vi "top_loop.vi"(0 "Input parameters":T4={"Measurement type"=enum."Debug", "Sensor type"=enum."HPK_8in_256", "Identifier"="test.txt", "Open after execution?"=FALSE, "Plot after execution?"=FALSE, "Display channel"=0, "Voltage Delay (s)"=0.5, "Switch Delay (s)"=0.01, "VISA resource name source"="", "VISA resource name DMM"="", "VISA resource name LCR"="", "Compliance  Level (A)"=10.0, "Voltage Limit (V)"=1000.0, "Data storage location"="", "Scan voltages"="", "Use source as DMM?"=FALSE, "LCR signal frequenzy (Hz)"=10.0, "DMM device"=enum."Keithley2001", "Sampling number"=1, "Use env. sensors on"=enum."Sensirion sht1x/7x", "Switchboard Handle"=0, "Use Switchboard"=FALSE, "LCR signal voltage (V)"=10000.0, "Repeat"=1, "Scan voltages IV"="", "Scan voltages CV"="", "Hex pad numbers?"=FALSE, "Set measurement type"=enum."Debug", "Custom pad scan"="", "IV voltage Delay (s)"=0.5, "CV voltage Delay (s)"=0.5, "Needle measurement?"=FALSE, "Comments"="test.txt", "LCR signal frequenzy (kHz)"=10.0, "Compliance  Level (uA)"=10.0, "Open Correction Array"=array2304x3[6912 elements], "Current set voltage"=0.0, "Last set voltage"=0.0, "Current channel"=0, "Last OpenCorrection index"=-1, "Total curr/vltg every x steps"=10, "Current channel iteration"=0, "No CV corrections"=FALSE, "Mapfile"="", "Corrfile"="", "IV voltage file"=path "", "CV voltage file"=path "", "IV Switch Delay (s)"=0.01, "CV Switch Delay (s)"=0.01, "Invert polarity"=FALSE, "Set debug dirs"=FALSE, "Is n on p"=FALSE} {"CV Switch Delay (s)" format="%#_13g"; "IV Switch Delay (s)" format="%#_13g"; "Last set voltage" format="%#_13g"; "Current set voltage" format="%#_13g"; "CV voltage Delay (s)" format="%#_13g"; "IV voltage Delay (s)" format="%#_13g"; "Voltage Limit (V)" format="%#_13g"; "Voltage Delay (s)" format="%#_13g"; "Switch Delay (s)" format="%#_13g"}, 5 "Dynamic data":T3, 7 "Front_panel_refs":T1, 11 "error in (no error)":errorcluster, 12 "Environmental data":T2) -> (4 "Input parameters out":T4={"Measurement type"=enum."Debug", "Sensor type"=enum."HPK_8in_256", "Identifier"="test.txt", "Open after execution?"=FALSE, "Plot after execution?"=FALSE, "Display channel"=0, "Voltage Delay (s)"=0.5, "Switch Delay (s)"=0.01, "VISA resource name source"="", "VISA resource name DMM"="", "VISA resource name LCR"="", "Compliance  Level (A)"=10.0, "Voltage Limit (V)"=1000.0, "Data storage location"="", "Scan voltages"="", "Use source as DMM?"=FALSE, "LCR signal frequenzy (Hz)"=10.0, "DMM device"=enum."Keithley2001", "Sampling number"=1, "Use env. sensors on"=enum."Sensirion sht1x/7x", "Switchboard Handle"=0, "Use Switchboard"=FALSE, "LCR signal voltage (V)"=10000.0, "Repeat"=1, "Scan voltages IV"="", "Scan voltages CV"="", "Hex pad numbers?"=FALSE, "Set measurement type"=enum."Debug", "Custom pad scan"="", "IV voltage Delay (s)"=0.5, "CV voltage Delay (s)"=0.5, "Needle measurement?"=FALSE, "Comments"="test.txt", "LCR signal frequenzy (kHz)"=10.0, "Compliance  Level (uA)"=10.0, "Open Correction Array"=array2304x3[6912 elements], "Current set voltage"=0.0, "Last set voltage"=0.0, "Current channel"=0, "Last OpenCorrection index"=-1, "Total curr/vltg every x steps"=10, "Current channel iteration"=0, "No CV corrections"=FALSE, "Mapfile"="", "Corrfile"="", "IV voltage file"=path "", "CV voltage file"=path "", "IV Switch Delay (s)"=0.01, "CV Switch Delay (s)"=0.01, "Invert polarity"=FALSE, "Set debug dirs"=FALSE, "Is n on p"=FALSE} {"CV Switch Delay (s)" format="%#_13g"; "IV Switch Delay (s)" format="%#_13g"; "Last set voltage" format="%#_13g"; "Current set voltage" format="%#_13g"; "CV voltage Delay (s)" format="%#_13g"; "IV voltage Delay (s)" format="%#_13g"; "Voltage Limit (V)" format="%#_13g"; "Voltage Delay (s)" format="%#_13g"; "Switch Delay (s)" format="%#_13g"}, 6 "Dynamic data out":T3, 8 "Front_panel_refs out":T1, 15 "error out":errorcluster)   [LabVIEW 2016]
doc: "The main loop function of the HexDAQ."
uses:
  <extravilib>/ChannelInstances/Tag-t'Env_data.ctl'.lvlib
  data_live.ctl
  input_params.ctl
  data_dynamic.ctl
  data_env.ctl
  <extravilib>/ChannelInstances/Tag-t'Env_data.ctl'/))Channel.ctl
  refs_front_panel.ctl
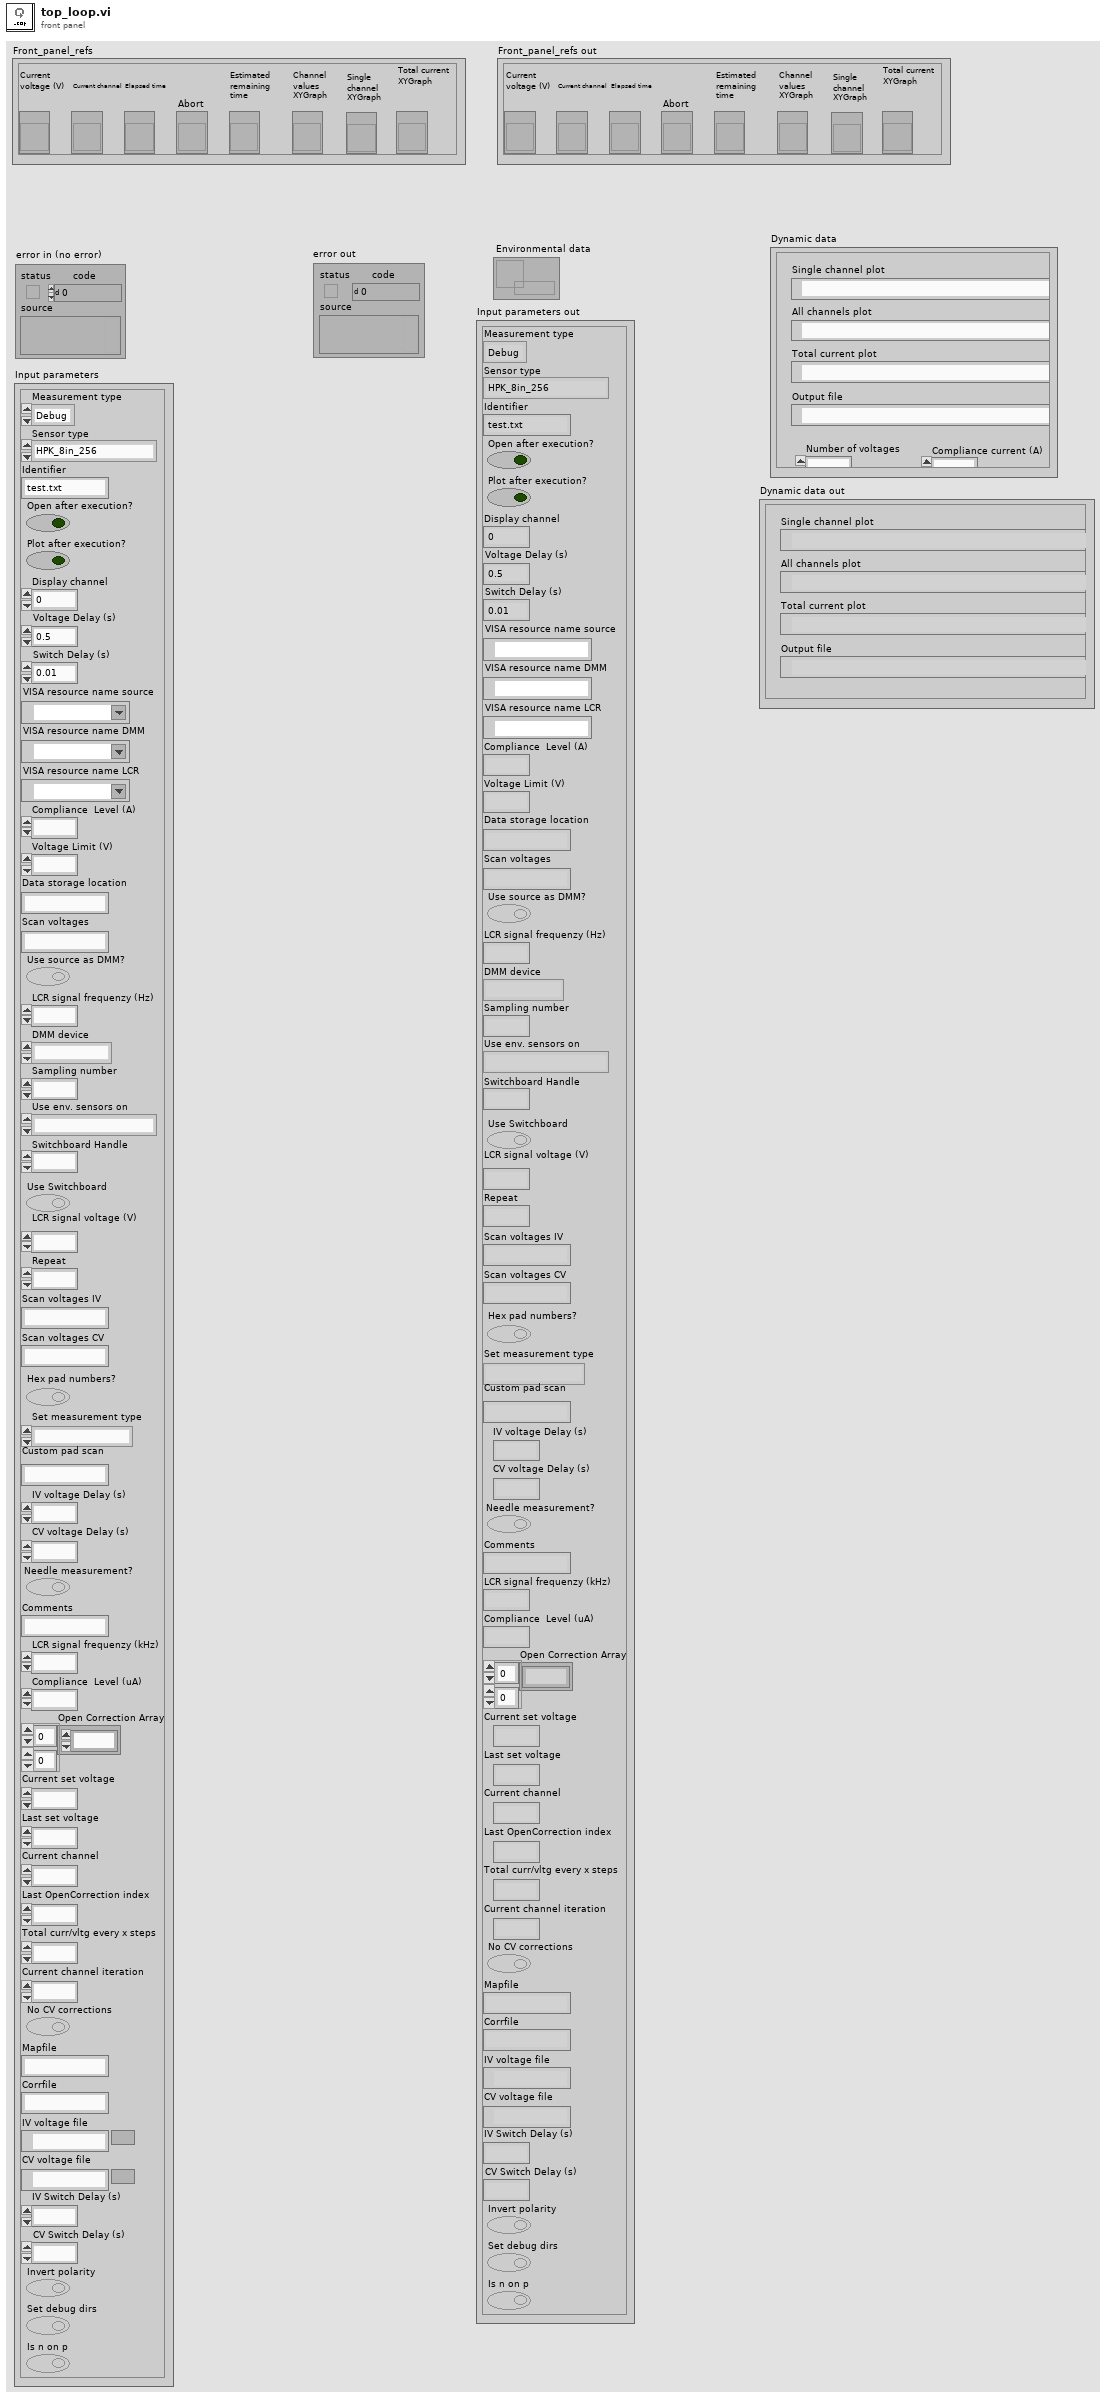
[diagram p1: front panel]
types:
  T1 = typedef "refs_front_panel.ctl" = cluster{"Current voltage (V)":refnum<vi>, "Elapsed time":refnum<vi>, "Current channel":refnum<vi>, "Abort":refnum<vi>, "Estimated remaining time":refnum<vi>, "Channel values XYGraph":refnum<vi>, "Single channel XYGraph":refnum<vi>, "Total current XYGraph":refnum<vi>}
  T2 = typedef "Tag-t'Env_data.ctl'.lvlib/))Channel.ctl" = refnum<queue>
  T3 = typedef "data_dynamic.ctl" = cluster{"Output file":path, "Y-label text":string, "Current set voltage":dbl, "Set voltage column":dbl[], "Pad number column":dbl[], "Data  column":dbl[], "Number of voltages":i32, "Compliance current (A)":dbl, "Geofile":string, "Peak voltage":dbl, "Hex PDF file":string, "Voltage array":dbl[], "Total current column":dbl[], "Timestamp column":dbl[], "Data name":string, "Data unit":string, "2nd data column":dbl[], "2nd data name":string, "2nd data unit":string, "3rd data column":dbl[], "4th data column":dbl[], "3rd data name":string, "3rd data unit":string, "4th data name":string, "4th data unit":string, "Actual voltage column":dbl[], "2nd Y-label text":string, "Single channel plot":path, "Temperature column":dbl[], "Humidity column":dbl[], "Channel switch array":i32[], "1st single plot name":string, "2nd single plot name":string, "All channels plot":path, "HexPlot command":string, "Custom channel array":i32[], "Data  error column":dbl[], "2nd data  error column":dbl[], "3rd data error column":dbl[], "4th data  error column":dbl[], "Total current plot":path, "5th data column":dbl[], "5th data  error column":dbl[], "6th data column":dbl[], "6th data  error column":dbl[], "5th data name":string, "5th data unit":string, "6th data name":string, "6th data unit":string, "HexPlot matrix command":string}
  T4 = typedef "input_params.ctl" = cluster{"Measurement type":enum16{"IV", "CV", "Debug", "Test_contact"}, "Sensor type":enum16{"HPK_6in_135", "HPK_8in_256", "IFX_8in_256", "Diode", "HPK_6in_256", "Full matrix"}, "Identifier":string, "Open after execution?":bool, "Plot after execution?":bool, "Display channel":i32, "Voltage Delay (s)":dbl, "Switch Delay (s)":dbl, "VISA resource name source":refnum<visa-resource-name>, "VISA resource name DMM":refnum<visa-resource-name>, "VISA resource name LCR":refnum<visa-resource-name>, "Compliance  Level (A)":dbl, "Voltage Limit (V)":dbl, "Data storage location":string, "Scan voltages":string, "Use source as DMM?":bool, "LCR signal frequenzy (Hz)":dbl, "DMM device":enum16{"Keithley2001", "Keithley2450", "Keithley2410", "Keithley6487"}, "Sampling number":i32, "Use env. sensors on":enum16{"Sensirion sht1x/7x", "Switch Matrix", "Probecard"}, "Switchboard Handle":u32, "Use Switchboard":bool, "LCR signal voltage (V)":dbl, "Repeat":i32, "Scan voltages IV":string, "Scan voltages CV":string, "Hex pad numbers?":bool, "Set measurement type":enum16{"IV", "CV", "Debug", "Test_contact", "IV+CV"}, "Custom pad scan":string, "IV voltage Delay (s)":dbl, "CV voltage Delay (s)":dbl, "Needle measurement?":bool, "Comments":string, "LCR signal frequenzy (kHz)":dbl, "Compliance  Level (uA)":dbl, "Open Correction Array":dbl[][], "Current set voltage":dbl, "Last set voltage":dbl, "Current channel":i32, "Last OpenCorrection index":i32, "Total curr/vltg every x steps":i32, "Current channel iteration":i32, "No CV corrections":bool, "Mapfile":string, "Corrfile":string, "IV voltage file":path, "CV voltage file":path, "IV Switch Delay (s)":dbl, "CV Switch Delay (s)":dbl, "Invert polarity":bool, "Set debug dirs":bool, "Is n on p":bool}
  T5 = typedef "data_live.ctl" = cluster{"Actual voltage":dbl, "Total current":dbl, "Data":dbl, "Data error":dbl, "2nd data":dbl, "2nd data error":dbl, "3rd data":dbl, "3rd data error":dbl, "4th data":dbl, "4th data error":dbl, "6th data error":dbl, "6th data":dbl, "5th data error":dbl, "5th data":dbl}
  T6 = enum16{"Sensirion sht1x/7x", "Switch Matrix", "Probecard"}
  T7 = typedef "data_env.ctl" = cluster{"Temp. Sensirion":dbl, "Hum. Sensirion":dbl, "Temp. Switch Matrix":dbl, "Hum. Switch Matrix":dbl, "Temp. Probecard":dbl, "Hum. Probecard":dbl}
  T8 = cluster{"XY Graph out":cluster{"Array":dbl[], "Array":dbl[]}[], "XY Graph out":cluster{"Array":dbl[], "Array":dbl[]}[]}
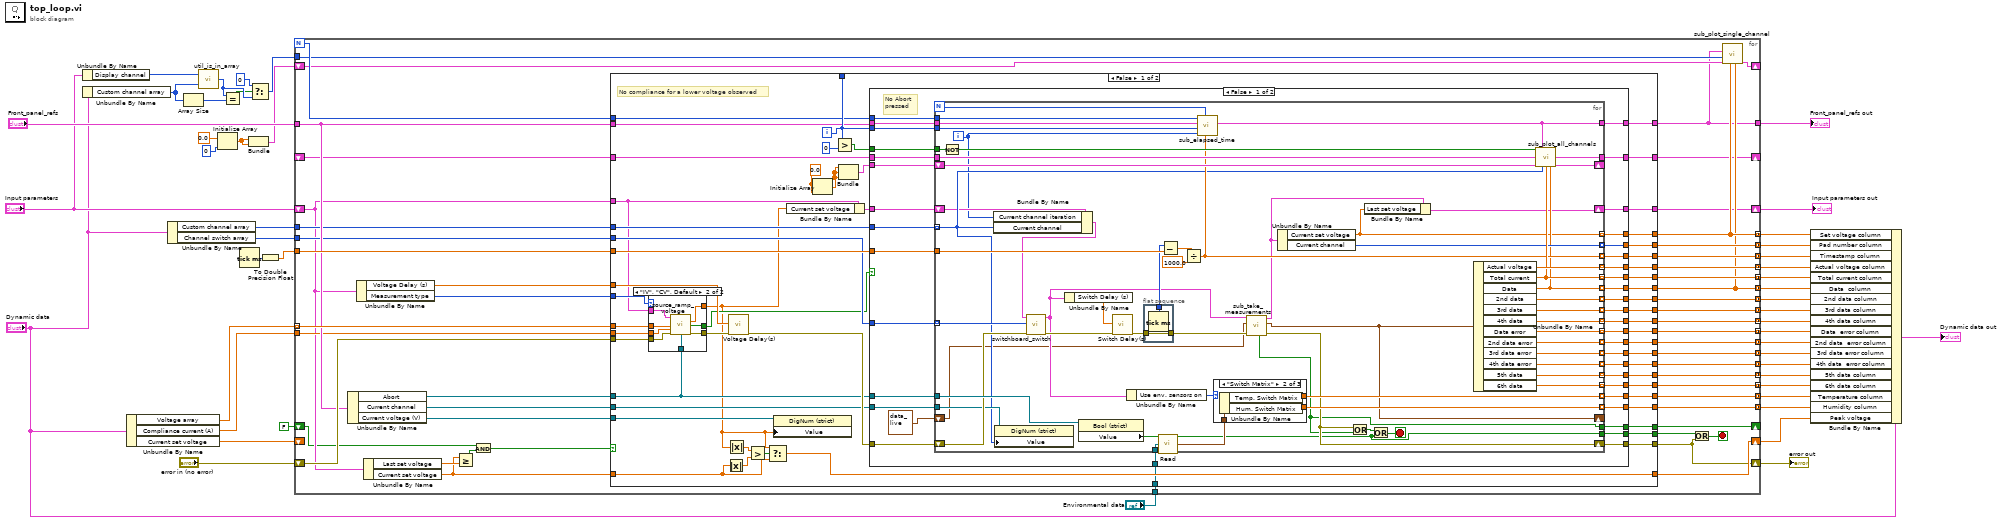
[diagram p0: block diagram]
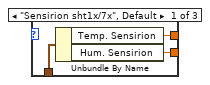
[diagram p2: hidden frame]
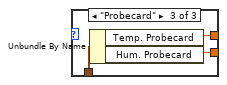
[diagram p3: hidden frame]
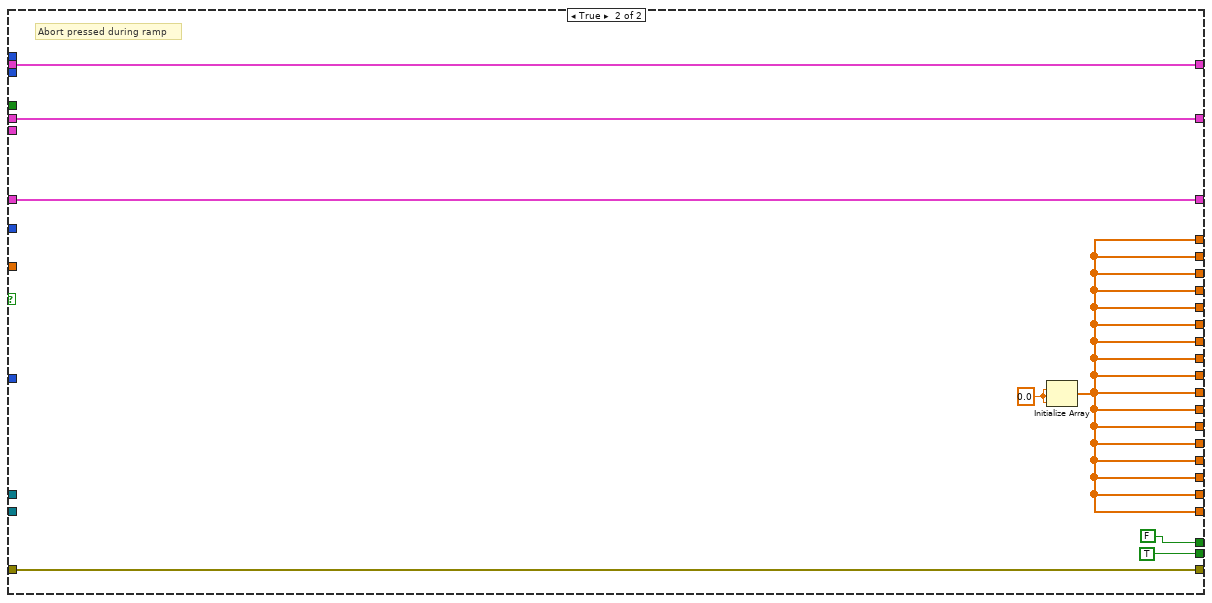
[diagram p4: hidden frame]
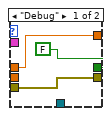
[diagram p5: hidden frame]
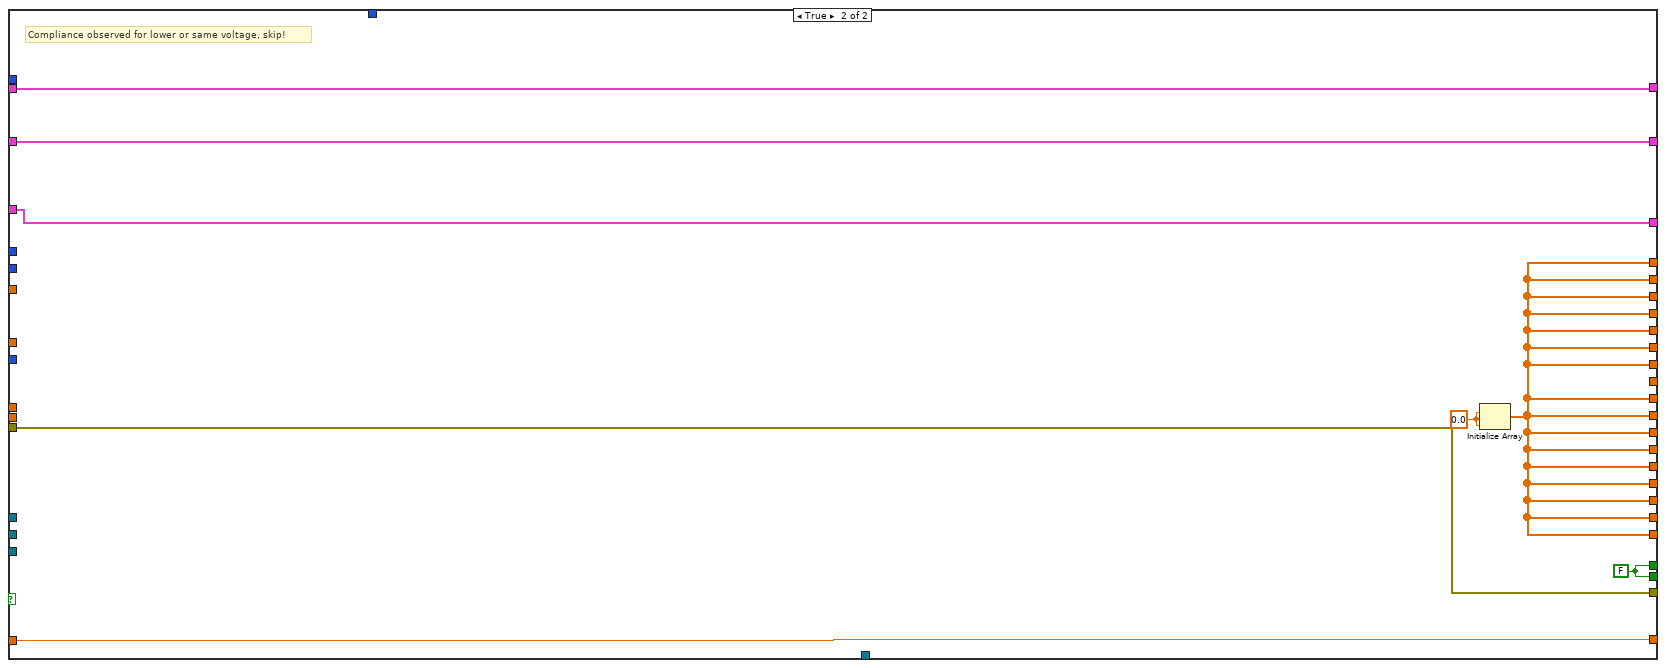
[diagram p6: hidden frame]
diagram:
  n1 = Unbundle By Name("Input parameters") -> ("Display channel"=w24:i32)
  n2 = Unbundle By Name("Dynamic data") -> ("Custom channel array"=w23:i32[])
  n3 = Unbundle By Name("Dynamic data") -> ("Voltage array"=w25:dbl[], "Compliance current (A)"=w2:dbl, "Current set voltage"=w10:dbl)
  n4 = Unbundle By Name("Dynamic data") -> ("Custom channel array"=w16:i32[], "Channel switch array"=w15:i32[])
  n5 = Array Size(array=w23) -> (size(s)=w19:i32)
  n6 = call "util_is_in_array.vi"("Array"=w23, "Numeric"=w24) -> ("Position"=w21:i32)
  n7 = Initialize Array(0.0 ("Secondary Parameter"), 0 ("dimension size")) -> (w12:dbl[])
  n8 = Equal?(x=w21, y=w19) -> (x = y?=w20:bool)
  n9 = Tick Count (ms)() -> (millisecond timer value=w27:u32)
  n10 = Bundle(w12, w12) -> (w11:cluster{dbl[], dbl[]})  [unwired: 1 in]
  n11 = Select(t=0, s=w20, f=w21) -> (s? t:f=w17:i32)
  n12 = To Double Precision Float(number=w27) -> (double precision float=w26:dbl)
  n13 = for {
    N -> [w85]
    tunnel: w25 -> [w92] mode=indexing
    tunnel: [w78] -> w7 mode=concatenating
    tunnel: [w77] -> w46 mode=concatenating
    tunnel: [w96] -> w6 mode=concatenating
    shift-right: [w57] -> w43
    shift-left: "error in (no error)" -> [w95]
    shift-right: [w70] -> w44
    shift-left: "Input parameters" -> [w54]
    tunnel: w26 -> [w89]
    shift-right: [w93] -> w38
    shift-left: w10 -> [_]
    tunnel: [w90] -> w8 mode=concatenating
    tunnel: [w88] -> w9 mode=concatenating
    tunnel: [w87] -> w42 mode=concatenating
    tunnel: [w84] -> w41 mode=concatenating
    tunnel: [w83] -> w40 mode=concatenating
    tunnel: [w82] -> w39 mode=concatenating
    tunnel: [w81] -> w37 mode=concatenating
    tunnel: [w80] -> w36 mode=concatenating
    tunnel: "Environmental data" -> [w79]
    tunnel: [w76] -> w32 mode=concatenating
    tunnel: [w75] -> w31 mode=concatenating
    tunnel: [w74] -> w30 mode=concatenating
    tunnel: [w73] -> w29 mode=concatenating
    tunnel: "Front_panel_refs" -> [w71]
    tunnel: w17 -> [w59]
    tunnel: w2 -> [w66]
    tunnel: w16 -> [w65]
    tunnel: w15 -> [w64]
    shift-right: [w63] -> _
    shift-left: _ -> [w62]
    shift-right: [w60] -> _
    shift-left: w11 -> [w61]
    tunnel: [w56] -> w5 mode=concatenating
    tunnel: [w55] -> w4 mode=concatenating
    tunnel: [w53] -> w3
    shift-right: [w52] -> _
    shift-left: FALSE ("Value") -> [w48]
    i -> [w86]
    stop <- w94 stop-if-true
    n14 = Unbundle By Name(w71) -> ("Abort"=w72:refnum<vi>, "Current channel"=w68:refnum<vi>, "Current voltage (V)"=w69:refnum<vi>)
    n15 = Unbundle By Name(w54) -> ("Voltage Delay (s)"=w67:dbl, "Measurement type"=w91:enum16{"IV", "CV", "Debug", "Test_contact"})
    n16 = Unbundle By Name(w54) -> ("Last set voltage"=w51:dbl, "Current set voltage"=w50:dbl)
    n17 = Greater Or Equal?(x=w50, y=w51) -> (x >= y?=w49:bool)
    n18 = And(x=w48, y=w49) -> (x .and. y?=w47:bool)
    n19 = case shown="False" w47 {
      tunnel: [w150 w283] -> w96
      tunnel: w95 -> [w149 w280]
      tunnel: [w146 w281] -> w93
      tunnel: w92 -> [w145 _]
      tunnel: w91 -> [w144 _]
      tunnel: [w142 w283] -> w90
      tunnel: w89 -> [w141 _]
      tunnel: [w140 w283] -> w88
      tunnel: [w139 w283] -> w87
      tunnel: w86 -> [w138 _]
      tunnel: w85 -> [w137 _]
      tunnel: [w136 _] -> w84
      tunnel: [w135 w283] -> w83
      tunnel: [w134 w283] -> w82
      tunnel: [w133 w283] -> w81
      tunnel: [w132 w283] -> w80
      tunnel: w79 -> [w131 _]
      tunnel: [w129 w283] -> w78
      tunnel: [w128 w283] -> w77
      tunnel: [w127 w283] -> w76
      tunnel: [w126 w283] -> w75
      tunnel: [w125 w283] -> w74
      tunnel: [w124 w283] -> w73
      tunnel: w72 -> [w123 _]
      tunnel: w71 -> [w122 w277]
      tunnel: [w121 w279] -> w70
      tunnel: w69 -> [w120 _]
      tunnel: w68 -> [w119 _]
      tunnel: w67 -> [w118 _]
      tunnel: w66 -> [w117 _]
      tunnel: w65 -> [w116 _]
      tunnel: w64 -> [w115 _]
      tunnel: [w112 w278] -> w63
      tunnel: w62 -> [w111 w278]
      tunnel: [w109 w282] -> w58
      tunnel: [w108 w280] -> w57
      tunnel: [w106 w283] -> w56
      tunnel: [w105 w283] -> w55
      tunnel: w54 -> [w100 w279]
      tunnel: [w99 w277] -> w53
      tunnel: [w98 w282] -> w52
      tunnel: w50 -> [w97 w281]
      frame False {
        w130 = 0.0 ("dimension size")
        # "No compliance for a lower voltage observed"
        n20 = case shown="\"IV\", \"CV\", Default" w144 {
          tunnel: w145 -> [w267 w274]
          tunnel: w149 -> [w268 w275]
          tunnel: [w268 w276] -> w148
          tunnel: w117 -> [_ w273]
          tunnel: [w267 w272] -> w101
          tunnel: w123 -> [_ w269]
          tunnel: [FALSE ("Aborted?") w271] -> w107
          tunnel: w100 -> [_ w270]
          frame "Debug" {
          }
          frame "IV", "CV", Default {
            n21 = call "source_ramp_voltage.vi"("Input parameters"=w270, "Target voltage (V)"=w274, "Compliance Current (A)"=w273, "error in (no error)"=w275, "Stop"=w269) -> ("Current voltage out (V)"=w272:dbl, "Aborted?"=w271:bool, "error out"=w276:errorcluster)  [unwired: 7 in, 1 out]
          }
        }
        n22 = Absolute Value(x=w97) -> (abs(x)=w102:dbl)
        n23 = Absolute Value(x=w101) -> (abs(x)=w103:dbl)
        n24 = call "Voltage Delay(s)"("error in (no error)"=w148, "Delay Time (s)"=w118) -> ("error out"=w143:errorcluster)  [unwired: 9 in]
        n25 = Greater?(x=w103, y=w102) -> (0:w104:bool)
        n26 = Select(t=w101, s=w104, f=w97) -> (s? t:f=w146:dbl)
        n27 = property class="DigNum (strict)"(reference=w120, "Value"=w101) -> ()  [unwired: 1 in, 2 out]
        n28 = Bundle By Name(cluster=w100, "Current set voltage"=w101) -> (w110:T4)
        n29 = Initialize Array(w130, w130) -> (w114:dbl[])
        n30 = Greater?(x=w138, y=0) -> (0:w147:bool)
        n31 = Bundle(w114, w114, w114) -> (w113:cluster{dbl[], dbl[], dbl[]})  [unwired: 1 in]
        n32 = case shown="False" w107 {
          tunnel: [w189 w260] -> w150
          tunnel: w147 -> [w188 _]
          tunnel: w143 -> [w187 w263]
          tunnel: [w186 w260] -> w142
          tunnel: w141 -> [w185 _]
          tunnel: [w184 w260] -> w140
          tunnel: [w183 w260] -> w139
          tunnel: w138 -> [w182 _]
          tunnel: w137 -> [w181 _]
          tunnel: [w180 w260] -> w136
          tunnel: [w179 w260] -> w135
          tunnel: [w178 w260] -> w134
          tunnel: [w177 w260] -> w133
          tunnel: [w176 w260] -> w132
          tunnel: w131 -> [w175 _]
          tunnel: [w174 w260] -> w129
          tunnel: [w173 w260] -> w128
          tunnel: [w172 w260] -> w127
          tunnel: [w171 w260] -> w126
          tunnel: [w170 w260] -> w125
          tunnel: [w169 w260] -> w124
          tunnel: w123 -> [w168 _]
          tunnel: w122 -> [w167 w259]
          tunnel: [w166 w265] -> w121
          tunnel: w119 -> [w165 _]
          tunnel: w116 -> [w164 _]
          tunnel: w115 -> [w163 _]
          tunnel: w113 -> [w162 _]
          tunnel: [w161 w264] -> w112
          tunnel: w111 -> [w160 w264]
          tunnel: w110 -> [w159 w265]
          tunnel: [w158 TRUE ("Value")] -> w109
          tunnel: [w157 w263] -> w108
          tunnel: [w156 w260] -> w105
          tunnel: [w155 w260] -> w106
          tunnel: [w153 w259] -> w99
          tunnel: [w152 FALSE ("Value")] -> w98
          frame False {
            # "No Abort\npressed"
            n33 = for {
              N -> [w210]
              tunnel: w163 -> [w231] mode=indexing
              tunnel: [w207] -> w189 mode=indexing
              tunnel: [w204] -> w173 mode=indexing
              tunnel: [w195] -> w174 mode=indexing
              shift-right: [w203] -> w157
              shift-left: w187 -> [w233]
              tunnel: w188 -> [w225]
              tunnel: [w201] -> w158
              tunnel: w168 -> [w246]
              tunnel: [w213] -> w186 mode=indexing
              tunnel: w185 -> [w245]
              tunnel: [w211] -> w184 mode=indexing
              tunnel: [w224] -> w183 mode=indexing
              tunnel: w182 -> [w218]
              tunnel: w181 -> [w209]
              tunnel: [w240] -> w180 mode=indexing
              tunnel: [w239] -> w179 mode=indexing
              tunnel: [w238] -> w178 mode=indexing
              tunnel: [w236] -> w177 mode=indexing
              tunnel: [w235] -> w176 mode=indexing
              tunnel: w175 -> [w234]
              tunnel: w164 -> [w208] mode=indexing
              tunnel: [w229] -> w172 mode=indexing
              tunnel: [w228] -> w171 mode=indexing
              tunnel: [w227] -> w170 mode=indexing
              tunnel: [w226] -> w169 mode=indexing
              tunnel: w165 -> [w221]
              tunnel: w167 -> [w217]
              shift-right: [w216] -> _
              shift-left: w162 -> [w212]
              tunnel: [w214] -> w161
              tunnel: w160 -> [w215]
              shift-right: [w197] -> w166
              shift-left: w159 -> [w206]
              tunnel: [w199] -> w156 mode=indexing
              tunnel: [w198] -> w155 mode=indexing
              shift-right: [w194] -> _
              shift-left: T5 {"Actual voltage"=0.0, "Total current"=0.0, "Data"=0.0, "Data error"=0.0, "2nd data"=0.0, "2nd data error"=0.0, "3rd data"=0.0, "3rd data error"=0.0, "4th data"=0.0, "4th data error"=0.0, "6th data error"=0.0, "6th data"=0.0, "5th data error"=0.0, "5th data"=0.0} ("Live data out") -> [w193]
              tunnel: [w191] -> w153
              tunnel: [w190] -> w152
              i -> [w192]
              stop <- w200 stop-if-true
              n34 = Not(x=w225) -> (.not. x?=w223:bool)
              n35 = Bundle By Name(cluster=w206, "Current channel iteration"=w192, "Current channel"=w208) -> (w205:T4)
              n36 = property on="Property Node" class="DigNum (strict)"(reference=w221, "Value"=w208) -> ()  [unwired: 1 in, 2 out]
              n37 = call "switchboard_switch.vi"("error in"=w233, "Channel"=w231, "Input parameters in"=w205) -> ("error out"=w232:errorcluster, "Input parameters out"=w219:T4)  [unwired: 7 in]
              n38 = Unbundle By Name(w219) -> ("Switch Delay (s)"=w222:dbl)
              n39 = property class="Bool (strict)"(reference=w246) -> ("Value"=w201:bool)  [unwired: 1 in, 2 out]
              n40 = call "Switch Delay(s)"("error in (no error)"=w232, "Delay Time (s)"=w222) -> ("error out"=w242:errorcluster)  [unwired: 9 in]
              n41 = Unbundle By Name(w219) -> ("Use env. sensors on"=w230:T6)
              n42 = flat-sequence {
                tunnel: [w257] -> w243
                tunnel: w242 -> [w256]
                tunnel: [w256] -> w241
                frame #0 {
                  n43 = Tick Count (ms)() -> (millisecond timer value=w257:u32)
                }
              }
              n44 = call <extravilib>:"Read.vi"("channel"=w234) -> ("element"=w237:T7)  [unwired: 1 in, 1 out]
              n45 = Subtract(x=w243, y=w245) -> (x-y=w220:dbl)
              n46 = Divide(x=w220, y=1000.0) -> (x/y=w211:dbl)
              n47 = call "sub_elapsed_time.vi"("Elapsed time (s)"=w211, "Inner N"=w210, "Inner i"=w192, "Outer i"=w218, "Front_panel_refs"=w217, "Outer N"=w209) -> ("Front_panel_refs out"=w191:T1)  [unwired: 5 in]
              n48 = case shown="\"Switch Matrix\"" w230 {
                tunnel: w237 -> [w249 w252 w255]
                tunnel: [w248 w250 w253] -> w236
                tunnel: [w247 w251 w254] -> w235
                frame "Sensirion sht1x/7x", Default {
                  n49 = Unbundle By Name(w249) -> ("Temp. Sensirion"=w248:dbl, "Hum. Sensirion"=w247:dbl)
                }
                frame "Switch Matrix" {
                  n50 = Unbundle By Name(w252) -> ("Temp. Switch Matrix"=w250:dbl, "Hum. Switch Matrix"=w251:dbl)
                }
                frame "Probecard" {
                  n51 = Unbundle By Name(w255) -> ("Temp. Probecard"=w253:dbl, "Hum. Probecard"=w254:dbl)
                }
              }
              n52 = call "sub_take_measurements.vi"("error in (no error)"=w241, "Live data in"=w193, "Input parameters"=w219) -> ("error out"=w203:errorcluster, "Live data out"=w194:T5, "Input parameters out"=w196:T4, "Compliance reached?"=w190:bool)  [unwired: 5 in]
              n53 = Unbundle By Name(w196) -> ("Current set voltage"=w195:dbl, "Current channel"=w207:i32)
              n54 = Or(x=w203, y=w190) -> (x .or. y?=w202:bool)
              n55 = Bundle By Name(cluster=w196, "Last set voltage"=w195) -> (w197:T4)
              n56 = Or(x=w202, y=w201) -> (x .or. y?=w200:bool)
              n57 = Unbundle By Name(w194) -> ("Actual voltage"=w238:dbl, "Total current"=w213:dbl, "Data"=w204:dbl, "2nd data"=w224:dbl, "3rd data"=w240:dbl, "4th data"=w239:dbl, "Data error"=w229:dbl, "2nd data error"=w228:dbl, "3rd data error"=w227:dbl, "4th data error"=w226:dbl, "5th data"=w199:dbl, "6th data"=w198:dbl)
              n58 = call "sub_plot_all_channels.vi"("Is first?"=w223, "Front_panel_refs"=w191, "Plot cluster"=w215, "Cluster"=w212, "Custom channel"=w208, "Total current"=w213, "Data"=w204) -> ("Plot cluster out"=w214:T8, "Cluster out"=w216:cluster{dbl[], dbl[], dbl[]})  [unwired: 7 in]
            }
          }
          frame True {
            w261 = 0.0 ("dimension size")
            # "Abort pressed during ramp"
            n59 = Initialize Array(w261, w261) -> (w260:dbl[])
          }
        }
      }
      frame True {
        w282 = FALSE ("Value")
        w284 = 0.0 ("dimension size")
        # "Compliance observed for lower or same voltage, skip!"
        n60 = Initialize Array(w284, w284) -> (w283:dbl[])
      }
    }
    n61 = Or(x=w58, y=w57) -> (x .or. y?=w94:bool)
    n62 = call "sub_plot_single_channel.vi"("Data column"=w77, "Set voltage column"=w78, "Cluster"=w61, "Channel"=w59, "Front_panel_refs"=w53) -> ("Cluster out"=w60:cluster{dbl[], dbl[]})  [unwired: 6 in]
  }
  "error out" <- w43
  "Input parameters out" <- w44
  "Front_panel_refs out" <- w3
  n63 = Bundle By Name(cluster="Dynamic data", "Set voltage column"=w7, "Pad number column"=w6, "Timestamp column"=w9, "Actual voltage column"=w39, "Total current column"=w8, "Data  column"=w46, "2nd data column"=w42, "3rd data column"=w41, "4th data column"=w40, "Data  error column"=w32, "2nd data  error column"=w31, "3rd data error column"=w30, "4th data  error column"=w29, "5th data column"=w4, "6th data column"=w5, "Temperature column"=w37, "Humidity column"=w36, "Peak voltage"=w38) -> (→"Dynamic data out":T3)
